vi "ROI Reference hs.vi"(8 "error in (no error)":errorcluster, 9 "Path":path, 10 "ROIs":T2={[0, 0, 2592, 1944], [{"Contour Type"=0, "ROI Type"=12, [85, 255, 293, 462, 89840]}, {"Contour Type"=0, "ROI Type"=12, [85, 463, 293, 670, 89840]}, {"Contour Type"=0, "ROI Type"=12, [84, 670, 292, 878, 89840]}, {"Contour Type"=0, "ROI Type"=12, [84, 878, 292, 1085, 89840]}, {"Contour Type"=0, "ROI Type"=12, [84, 1086, 292, 1290, 89840]}, {"Contour Type"=0, "ROI Type"=12, [84, 1294, 292, 1501, 89840]}, {"Contour Type"=0, "ROI Type"=12, [84, 1502, 292, 1708, 89840]}, {"Contour Type"=0, "ROI Type"=12, [83, 1709, 291, 1916, 89840]}, {"Contour Type"=0, "ROI Type"=12, [294, 256, 502, 463, 89840]}, {"Contour Type"=0, "ROI Type"=12, [293, 463, 501, 670, 89840]}, {"Contour Type"=0, "ROI Type"=12, [293, 671, 501, 878, 89840]}, {"Contour Type"=0, "ROI Type"=12, [293, 879, 501, 1086, 89840]}, {"Contour Type"=0, "ROI Type"=12, [293, 1087, 501, 1294, 89840]}, {"Contour Type"=0, "ROI Type"=12, [292, 1294, 500, 1501, 89840]}, {"Contour Type"=0, "ROI Type"=12, [292, 1502, 500, 1709, 89840]}, {"Contour Type"=0, "ROI Type"=12, [292, 1710, 500, 1917, 89840]}, {"Contour Type"=0, "ROI Type"=12, [502, 256, 710, 463, 89840]}, {"Contour Type"=0, "ROI Type"=12, [502, 464, 710, 671, 89840]}, {"Contour Type"=0, "ROI Type"=12, [502, 672, 710, 879, 89840]}, {"Contour Type"=0, "ROI Type"=12, [502, 879, 710, 1086, 89840]}, {"Contour Type"=0, "ROI Type"=12, [501, 1087, 709, 1294, 89840]}, {"Contour Type"=0, "ROI Type"=12, [501, 1295, 709, 1502, 89840]}, {"Contour Type"=0, "ROI Type"=12, [501, 1503, 709, 1710, 89840]}, {"Contour Type"=0, "ROI Type"=12, [501, 1710, 709, 1917, 89840]}, {"Contour Type"=0, "ROI Type"=12, [711, 257, 919, 464, 89840]}, {"Contour Type"=0, "ROI Type"=12, [711, 464, 919, 672, 89840]}, {"Contour Type"=0, "ROI Type"=12, [710, 672, 918, 879, 89840]}, {"Contour Type"=0, "ROI Type"=12, [710, 880, 918, 1087, 89840]}, {"Contour Type"=0, "ROI Type"=12, [710, 1088, 918, 1295, 89840]}, {"Contour Type"=0, "ROI Type"=12, [710, 1296, 918, 1502, 89840]}, {"Contour Type"=0, "ROI Type"=12, [710, 1503, 918, 1710, 89840]}, {"Contour Type"=0, "ROI Type"=12, [709, 1711, 917, 1918, 89840]}, {"Contour Type"=0, "ROI Type"=12, [920, 257, 1128, 464, 89840]}, {"Contour Type"=0, "ROI Type"=12, [919, 465, 1127, 672, 89840]}, {"Contour Type"=0, "ROI Type"=12, [919, 673, 1127, 880, 89840]}, {"Contour Type"=0, "ROI Type"=12, [919, 881, 1127, 1088, 89840]}, {"Contour Type"=0, "ROI Type"=12, [919, 1088, 1127, 1295, 89840]}, {"Contour Type"=0, "ROI Type"=12, [918, 1296, 1126, 1503, 89840]}, {"Contour Type"=0, "ROI Type"=12, [918, 1504, 1126, 1711, 89840]}, {"Contour Type"=0, "ROI Type"=12, [918, 1712, 1126, 1919, 89840]}, {"Contour Type"=0, "ROI Type"=12, [1128, 258, 1336, 465, 89840]}, {"Contour Type"=0, "ROI Type"=12, [1128, 466, 1336, 673, 89840]}, {"Contour Type"=0, "ROI Type"=12, [1128, 673, 1336, 880, 89840]}, {"Contour Type"=0, "ROI Type"=12, [1128, 881, 1336, 1088, 89840]}, {"Contour Type"=0, "ROI Type"=12, [1127, 1089, 1335, 1296, 89840]}, {"Contour Type"=0, "ROI Type"=12, [1127, 1297, 1335, 1504, 89840]}, {"Contour Type"=0, "ROI Type"=12, [1127, 1504, 1335, 1711, 89840]}, {"Contour Type"=0, "ROI Type"=12, [1127, 1712, 1335, 1919, 89840]}, {"Contour Type"=0, "ROI Type"=12, [1337, 258, 1545, 466, 89840]}, {"Contour Type"=0, "ROI Type"=12, [1337, 466, 1545, 673, 89840]}, {"Contour Type"=0, "ROI Type"=12, [1336, 674, 1544, 881, 89840]}, {"Contour Type"=0, "ROI Type"=12, [1336, 882, 1544, 1089, 89840]}, {"Contour Type"=0, "ROI Type"=12, [1336, 1090, 1544, 1296, 89840]}, {"Contour Type"=0, "ROI Type"=12, [1336, 1297, 1544, 1504, 89840]}, {"Contour Type"=0, "ROI Type"=12, [1336, 1505, 1544, 1712, 89840]}, {"Contour Type"=0, "ROI Type"=12, [1335, 1713, 1543, 1920, 89840]}, {"Contour Type"=0, "ROI Type"=12, [1546, 259, 1754, 466, 89840]}, {"Contour Type"=0, "ROI Type"=12, [1545, 467, 1753, 674, 89840]}, {"Contour Type"=0, "ROI Type"=12, [1545, 675, 1753, 882, 89840]}, {"Contour Type"=0, "ROI Type"=12, [1545, 882, 1753, 1089, 89840]}, {"Contour Type"=0, "ROI Type"=12, [1545, 1090, 1753, 1297, 89840]}, {"Contour Type"=0, "ROI Type"=12, [1544, 1298, 1752, 1505, 89840]}, {"Contour Type"=0, "ROI Type"=12, [1544, 1506, 1752, 1713, 89840]}, {"Contour Type"=0, "ROI Type"=12, [1544, 1713, 1752, 1920, 89840]}, {"Contour Type"=0, "ROI Type"=12, [1754, 260, 1962, 467, 89840]}, {"Contour Type"=0, "ROI Type"=12, [1754, 467, 1962, 674, 89840]}, {"Contour Type"=0, "ROI Type"=12, [1754, 675, 1962, 882, 89840]}, {"Contour Type"=0, "ROI Type"=12, [1754, 883, 1962, 1090, 89840]}, {"Contour Type"=0, "ROI Type"=12, [1753, 1091, 1961, 1298, 89840]}, {"Contour Type"=0, "ROI Type"=12, [1753, 1298, 1961, 1505, 89840]}, {"Contour Type"=0, "ROI Type"=12, [1753, 1506, 1961, 1713, 89840]}, {"Contour Type"=0, "ROI Type"=12, [1753, 1714, 1961, 1921, 89840]}, {"Contour Type"=0, "ROI Type"=12, [1963, 260, 2171, 467, 89840]}, {"Contour Type"=0, "ROI Type"=12, [1963, 468, 2171, 675, 89840]}, {"Contour Type"=0, "ROI Type"=12, [1962, 676, 2170, 883, 89840]}, {"Contour Type"=0, "ROI Type"=12, [1962, 884, 2170, 1090, 89840]}, {"Contour Type"=0, "ROI Type"=12, [1962, 1091, 2170, 1298, 89840]}, {"Contour Type"=0, "ROI Type"=12, [1962, 1299, 2170, 1506, 89840]}, {"Contour Type"=0, "ROI Type"=12, [1962, 1507, 2170, 1714, 89840]}, {"Contour Type"=0, "ROI Type"=12, [1961, 1714, 2169, 1922, 89840]}, {"Contour Type"=0, "ROI Type"=12, [2172, 261, 2380, 468, 89840]}, {"Contour Type"=0, "ROI Type"=12, [2171, 469, 2379, 676, 89840]}, {"Contour Type"=0, "ROI Type"=12, [2171, 676, 2379, 883, 89840]}, {"Contour Type"=0, "ROI Type"=12, [2171, 884, 2379, 1091, 89840]}, {"Contour Type"=0, "ROI Type"=12, [2171, 1092, 2379, 1299, 89840]}, {"Contour Type"=0, "ROI Type"=12, [2170, 1300, 2378, 1507, 89840]}, {"Contour Type"=0, "ROI Type"=12, [2170, 1507, 2378, 1714, 89840]}, {"Contour Type"=0, "ROI Type"=12, [2170, 1715, 2378, 1922, 89840]}, {"Contour Type"=0, "ROI Type"=12, [2380, 261, 2588, 468, 89840]}, {"Contour Type"=0, "ROI Type"=12, [2380, 469, 2588, 676, 89840]}, {"Contour Type"=0, "ROI Type"=12, [2380, 677, 2588, 884, 89840]}, {"Contour Type"=0, "ROI Type"=12, [2380, 885, 2588, 1092, 89840]}, {"Contour Type"=0, "ROI Type"=12, [2379, 1092, 2587, 1299, 89840]}, {"Contour Type"=0, "ROI Type"=12, [2379, 1300, 2587, 1507, 89840]}, {"Contour Type"=0, "ROI Type"=12, [2379, 1508, 2587, 1715, 89840]}, {"Contour Type"=0, "ROI Type"=12, [2379, 1716, 2587, 1923, 89840]}]}, 11 "queue name":string="display1") -> (0 "error out":errorcluster)   [LabVIEW 2019]
panel:
  in  "Font, Size & Style":T1={"Desired Font (Application)"=enum."Application Font", "[User-specified Font]"={"Font Name"="", "Size"=12, "Strikeout?"=FALSE, "Italic?"=FALSE, "Underline?"=FALSE, "Outline?"=FALSE, "Shadow?"=FALSE, "Bold?"=FALSE, "Rotation Angle"=0.0}, "Horizontal Alignment"=0, "Vertical Alignment"=0} {"Vertical Alignment" items=["Bottom", "Top", "Baseline"]; "Horizontal Alignment" items=["Left", "Center", "Right"]; "[User-specified Font]"."Rotation Angle" format="%.2f"}
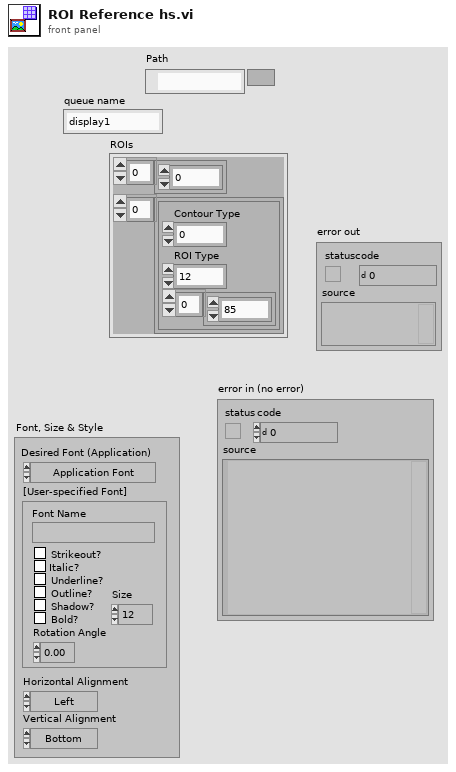
[diagram p1: front panel]
types:
  T1 = cluster{"Desired Font (Application)":enum16{"User-specified Font", "Application Font", "System Font", "Dialog Font"}, "[User-specified Font]":cluster{"Font Name":string, "Size":i16, "Strikeout?":bool, "Italic?":bool, "Underline?":bool, "Outline?":bool, "Shadow?":bool, "Bold?":bool, "Rotation Angle":dbl}, "Horizontal Alignment":i16, "Vertical Alignment":i16}
  T2 = cluster{i32[], cluster{"Contour Type":u32, "ROI Type":u32, i32[]}[]}
  T3 = typedef "Image Type" = u32
  T4 = typedef "IMAQ Image.ctl" = refnum<image>
  T5 = cluster{"Contour Type":u32, "ROI Type":u32, i32[]}[]
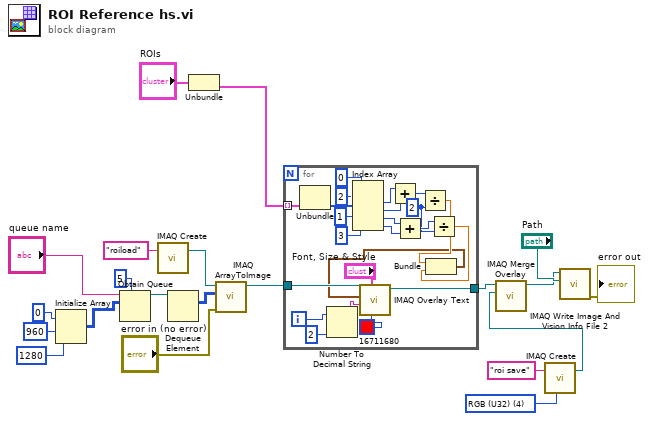
[diagram p0: block diagram]
diagram:
  w6 = T3 4 items=["Grayscale (U8)", "Grayscale (I16)", "Grayscale (SGL)", "Complex (CSG)", "RGB (U32)", "HSL (U32)", "RGB (U64)", "Grayscale (U16)"] ("Image Type")
  n1 = Initialize Array(u8 0 ("element"), 960 ("dimension size"), 1280 ("dimension size")) -> (w14:u8[][])
  n2 = Obtain Queue(max queue size (-1, unlimited)=5, name (unnamed)="queue name", element data type=w14) -> (queue out=w13:refnum<queue>)  [unwired: 2 in, 2 out]
  n3 = call "IMAQ Create"("Image Name"="roiload") -> ("New Image"=w20:T4)  [unwired: 4 in, 1 out]
  n4 = Dequeue Element(queue=w13) -> (element=w12:u8[][])  [unwired: 2 in, 3 out]
  n5 = Unbundle("ROIs") -> (w10:T5)  [unwired: 1 out]
  n6 = call "IMAQ ArrayToImage"("error in (no error)"="error in (no error)", "Image Pixels (U8)"=w12, "Image"=w20) -> ("Image Out"=w9:T4)  [unwired: 7 in, 1 out]
  n7 = for {
    tunnel: w10 -> [w42] mode=indexing
    tunnel: w9 -> [w43]
    tunnel: [w22] -> w1
    i -> [w38]
    w28 = 2 ("y")
    n8 = Unbundle(w42) -> (w41:i32[])  [unwired: 2 out]
    n9 = Number To Decimal String(number=w38, width (-)=i16 2) -> (decimal integer string=w37:string)
    n10 = Index Array(array=w41, index #1=0 ("index"), index #2=2 ("index"), index #3=1 ("index"), index #4=3 ("index")) -> (element #1=w34:i32, element #2=w33:i32, element #3=w32:i32, element #4=w31:i32)
    n11 = Add(x=w34, y=w33) -> (x+y=w30:i32)
    n12 = Add(x=w32, y=w31) -> (x+y=w29:i32)
    n13 = Divide(x=w30, y=w28) -> (x/y=w27:dbl)
    n14 = Divide(x=w29, y=w28) -> (x/y=w26:dbl)
    n15 = Bundle(w27, w26) -> (w25:cluster{dbl, dbl})  [unwired: 1 in]
    n16 = call "IMAQ Overlay Text"("Text Color (black)"=u32 16711680, "Font, Size & Style"="Font, Size & Style", "String"=w37, "Origin"=w25, "Image"=w43) -> ("Image Out"=w22:T4)  [unwired: 5 in, 1 out]
  }
  n17 = call "IMAQ Create"("Image Name"="roi save", "Image Type"=w6) -> ("New Image"=w5:T4)  [unwired: 3 in, 1 out]
  n18 = call "IMAQ Merge Overlay"("Image Dst"=w5, "Image Src"=w1) -> ("Image Dst Out"=w2:T4)  [unwired: 8 in, 1 out]
  n19 = call "IMAQ Write Image And Vision Info File 2"("File Path"="Path", "Image"=w2) -> ("error out"=→"error out":errorcluster)  [unwired: 8 in, 1 out]
